vi "Scan_Percent.vi"(0 "开始时间":dbl, 1 "测量总数":dbl, 2 "当前索引":dbl, 3 "Error In":errorcluster caption="错误输入") -> (7 "当前进度(%)":dbl, 8 "当前进度":string, 10 "Error Out":errorcluster caption="错误输出")   [LabVIEW 2020]
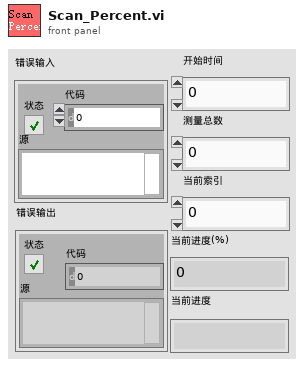
[diagram p1: front panel]
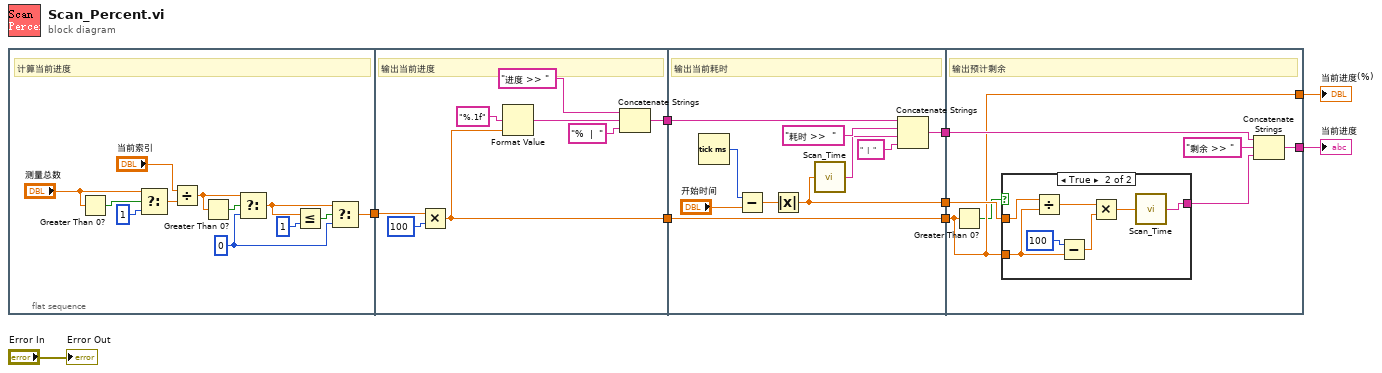
[diagram p0: block diagram]
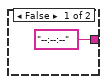
[diagram p2: hidden frame]
diagram:
  n1 = flat-sequence {
    tunnel: [w10] -> w7
    tunnel: w7 -> [w28]
    tunnel: [w23] -> w6
    tunnel: [w22] -> w5
    tunnel: w6 -> [w39]
    tunnel: [w39] -> w4
    tunnel: [w35] -> w3
    tunnel: w5 -> [w34]
    tunnel: [w30] -> w2
    tunnel: [w42] -> w9
    tunnel: w4 -> [w42]
    tunnel: w3 -> [w46]
    tunnel: w2 -> [w45]
    tunnel: [w40] -> w8
    frame #0 {
      w11 = 0
      # "计算当前进度"
      n2 = Greater Than 0?(x="测量总数") -> (x > 0?=w21:bool)
      n3 = Select(t="测量总数", s=w21, f=1) -> (s? t:f=w18:dbl)
      n4 = Divide(x="当前索引", y=w18) -> (x/y=w15:dbl)
      n5 = Greater Than 0?(x=w15) -> (x > 0?=w16:bool)
      n6 = Select(t=w15, s=w16, f=w11) -> (s? t:f=w12:dbl)
      n7 = Less Or Equal?(x=w12, y=1) -> (x <= y?=w13:bool)
      n8 = Select(t=w12, s=w13, f=w11) -> (s? t:f=w10:dbl)
    }
    frame #1 {
      # "输出当前进度"
      n9 = Multiply(x=w28, y=100) -> (x*y=w23:dbl)
      n10 = Format Value(format string="%.1f", value (0)=w23) -> (output string=w25:string)  [unwired: 1 in]
      n11 = Concatenate Strings("进度 >> ", w25, "%  |  ") -> (w22:string)
    }
    frame #2 {
      # "输出当前耗时"
      n12 = Tick Count (ms)() -> (millisecond timer value=w36:u32)
      n13 = Subtract(x=w36, y="开始时间") -> (x-y=w38:dbl)
      n14 = Absolute Value(x=w38) -> (abs(x)=w35:dbl)
      n15 = call "Scan_Time.vi"("时间差(ms)"=w35) -> ("时间字符串"=w32:string)
      n16 = Concatenate Strings(w34, "耗时 >>  ", w32, "  |  ") -> (w30:string)
    }
    frame #3 {
      # "输出预计剩余"
      n17 = Greater Than 0?(x=w42) -> (x > 0?=w41:bool)
      n18 = case shown="True" w41 {
        tunnel: w42 -> [_ w53]
        tunnel: w46 -> [_ w49]
        tunnel: ["--:--:--" w48] -> w43
        frame False {
        }
        frame True {
          n19 = Divide(x=w49, y=w53) -> (x/y=w52:dbl)
          n20 = Subtract(x=100, y=w53) -> (x-y=w51:dbl)
          n21 = Multiply(x=w52, y=w51) -> (x*y=w50:dbl)
          n22 = call "Scan_Time.vi"("时间差(ms)"=w50) -> ("时间字符串"=w48:string)
        }
      }
      n23 = Concatenate Strings(w45, "剩余 >> ", w43) -> (w40:string)
    }
  }
  "当前进度(%)" <- w9
  "当前进度" <- w8
  "Error Out" <- "Error In"
